vi "exercice7-3.vi"() -> ()   [LabVIEW 2013]
uses:
  <vilib>/Utility/file.llb/Write To Spreadsheet File (DBL).vi
  <vilib>/measure/NI_MABase.lvlib
panel:
  out "tableau ajouté":dbl[][](array[numeric])
  in  "nom du fichier":string
  out "Graphe":waveform(dbl)[](graph)
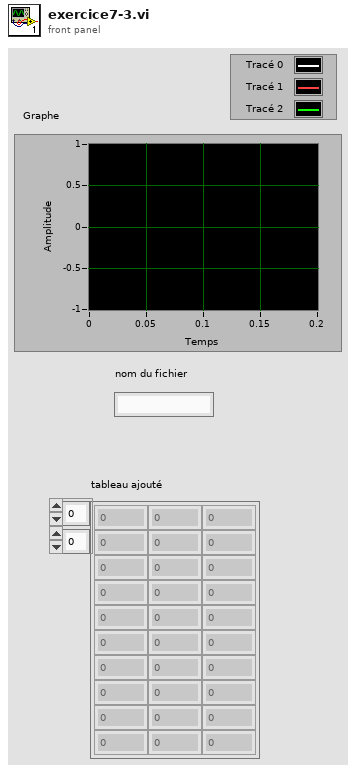
[diagram p1: front panel]
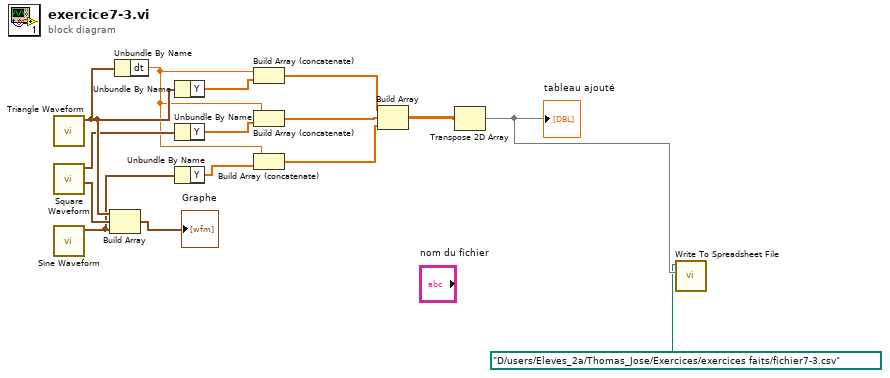
[diagram p0: block diagram]
diagram:
  n1 = call <vilib>:"Triangle Waveform.vi"() -> ("signal out"=w13:waveform(dbl))  [unwired: 10 in, 1 out]
  n2 = call <vilib>:"Square Waveform.vi"() -> ("signal out"=w12:waveform(dbl))  [unwired: 10 in, 1 out]
  n3 = call <vilib>:"Sine Waveform.vi"() -> ("signal out"=w11:waveform(dbl))  [unwired: 10 in, 1 out]
  n4 = Build Array(w13, w12, w11) -> (→"Graphe":waveform(dbl)[])
  n5 = Unbundle By Name(w13) -> ("dt"=w8:dbl)
  n6 = Unbundle By Name(w13) -> ("Y"=w10:dbl[])
  n7 = Unbundle By Name(w12) -> ("Y"=w9:dbl[])
  n8 = Unbundle By Name(w11) -> ("Y"=w7:dbl[])
  n9 = Build Array (concatenate)(w8, w10) -> (w6:dbl[])
  n10 = Build Array (concatenate)(w8, w9) -> (w5:dbl[])
  n11 = Build Array (concatenate)(w8, w7) -> (w4:dbl[])
  n12 = Build Array(w6, w5, w4) -> (w3:dbl[][])
  n13 = Transpose 2D Array(2D array=w3) -> (transposed array=w2:dbl[][])
  "tableau ajouté" <- w2
  n14 = call-poly <vilib>:"Write To Spreadsheet File.vi"("2D data"=w2, "file path (dialog if empty)"=path "D:/users/Eleves_2a/Thomas_Jose/Exercices/exercices faits/fichier7-3.csv") -> ()  [unwired: 6 in, 1 out]
